vi "DSOpen.vi"(8 "Array":string[](array[string]), 9 "mode":T1(ring), 10 "I/O":enum16{"Input", "Output"}(ring), 11 "Slot":T2(ring)=enum."Dnet1") -> (0 "error Out":errorcluster[](array[cluster]), 3 "connection out":refnum<k13>[](array[refnum]))   [LabVIEW 2011]
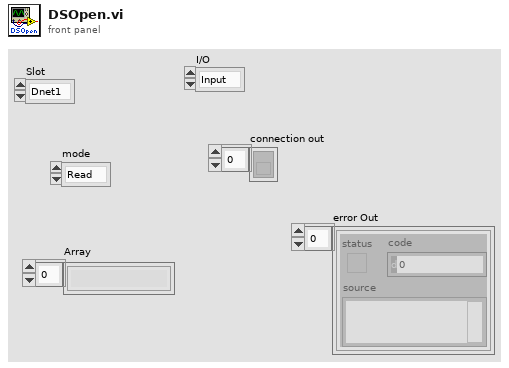
[diagram p1: front panel]
types:
  T1 = enum16{"Read", "Write", "ReadWrite", "BufferedRead", "BufferedReadWrite"}
  T2 = enum16{"OPC Server", "Global", "Dnet1", "Dnet2", "Dnet3", "Ain1", "Ain2", "Aout1", "Din1", "Din2", "Dout1"}
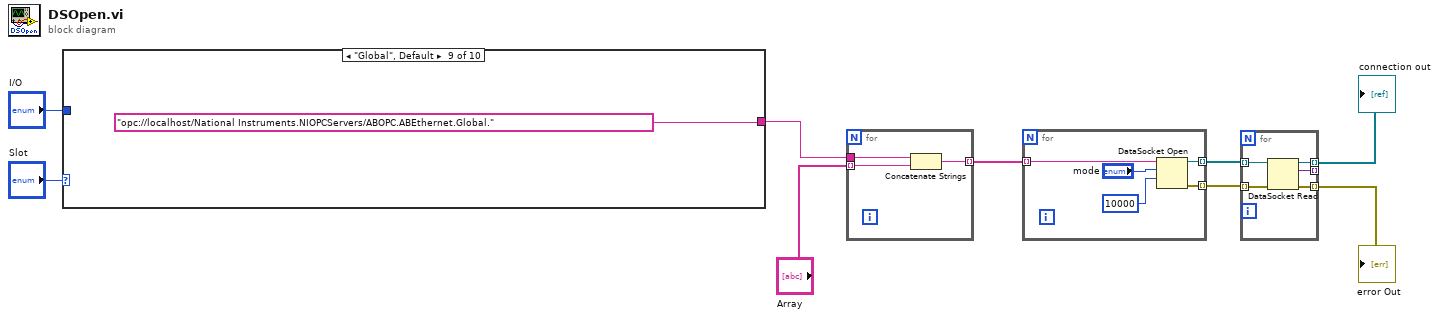
[diagram p0: block diagram]
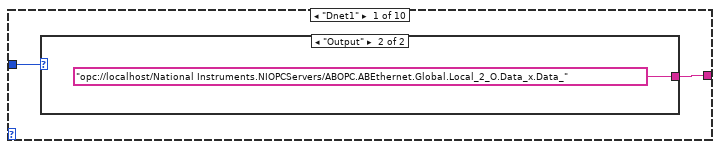
[diagram p2: hidden frame]
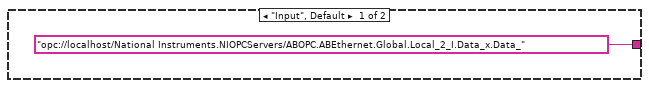
[diagram p3: hidden frame]
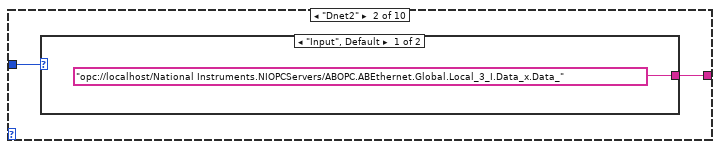
[diagram p4: hidden frame]
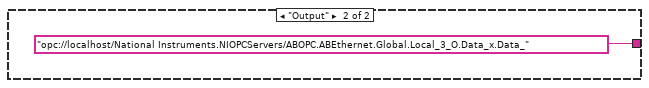
[diagram p5: hidden frame]
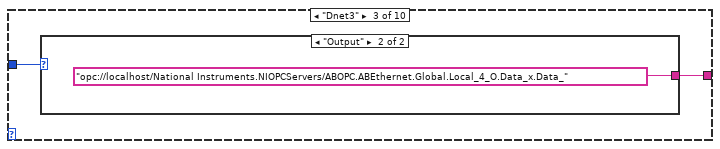
[diagram p6: hidden frame]
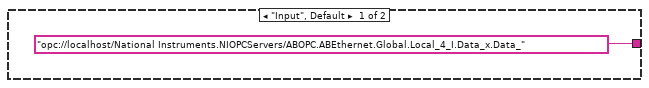
[diagram p7: hidden frame]
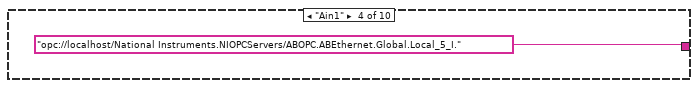
[diagram p8: hidden frame]
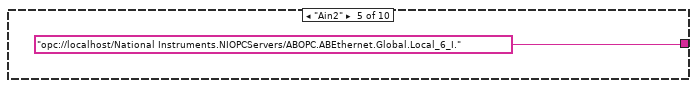
[diagram p9: hidden frame]
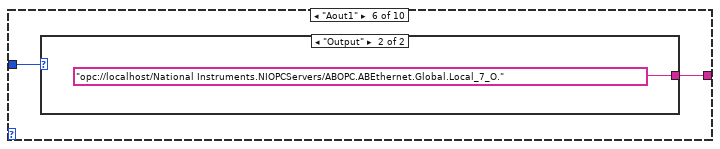
[diagram p10: hidden frame]
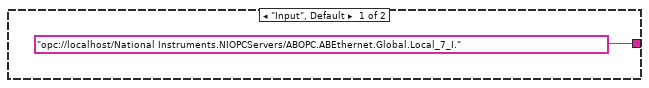
[diagram p11: hidden frame]
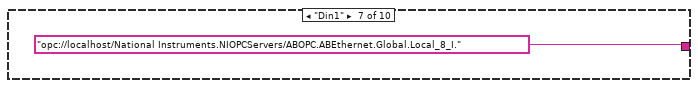
[diagram p12: hidden frame]
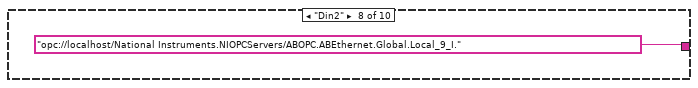
[diagram p13: hidden frame]
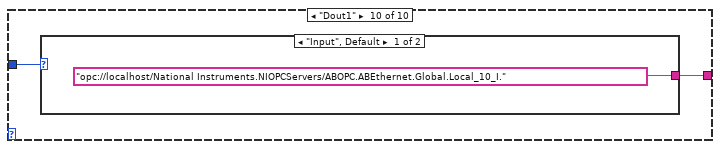
[diagram p14: hidden frame]
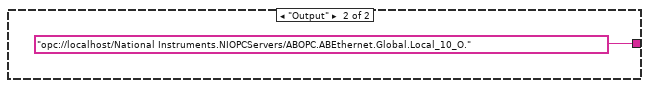
[diagram p15: hidden frame]
diagram:
  n1 = case shown="\"Global\", Default" "Slot" {
    tunnel: "I/O" -> [w11 w15 w19 _ _ w25 _ _ _ w32]
    tunnel: [w10 w14 w18 "opc://localhost/National Instruments.NIOPCServers/ABOPC.ABEthernet.Global.Local_5_I." "opc://localhost/National Instruments.NIOPCServers/ABOPC.ABEthernet.Global.Local_6_I." w24 "opc://localhost/National Instruments.NIOPCServers/ABOPC.ABEthernet.Global.Local_8_I." "opc://localhost/National Instruments.NIOPCServers/ABOPC.ABEthernet.Global.Local_9_I." "opc://localhost/National Instruments.NIOPCServers/ABOPC.ABEthernet.Global." w31] -> w8
    frame "Dnet1" {
      n2 = case shown="\"Output\"" w11 {
        tunnel: ["opc://localhost/National Instruments.NIOPCServers/ABOPC.ABEthernet.Global.Local_2_I.Data_x.Data_" "opc://localhost/National Instruments.NIOPCServers/ABOPC.ABEthernet.Global.Local_2_O.Data_x.Data_"] -> w10
        frame "Input", Default {
        }
        frame "Output" {
        }
      }
    }
    frame "Dnet2" {
      n3 = case shown="\"Input\", Default" w15 {
        tunnel: ["opc://localhost/National Instruments.NIOPCServers/ABOPC.ABEthernet.Global.Local_3_I.Data_x.Data_" "opc://localhost/National Instruments.NIOPCServers/ABOPC.ABEthernet.Global.Local_3_O.Data_x.Data_"] -> w14
        frame "Input", Default {
        }
        frame "Output" {
        }
      }
    }
    frame "Dnet3" {
      n4 = case shown="\"Output\"" w19 {
        tunnel: ["opc://localhost/National Instruments.NIOPCServers/ABOPC.ABEthernet.Global.Local_4_I.Data_x.Data_" "opc://localhost/National Instruments.NIOPCServers/ABOPC.ABEthernet.Global.Local_4_O.Data_x.Data_"] -> w18
        frame "Input", Default {
        }
        frame "Output" {
        }
      }
    }
    frame "Ain1" {
    }
    frame "Ain2" {
    }
    frame "Aout1" {
      n5 = case shown="\"Output\"" w25 {
        tunnel: ["opc://localhost/National Instruments.NIOPCServers/ABOPC.ABEthernet.Global.Local_7_I." "opc://localhost/National Instruments.NIOPCServers/ABOPC.ABEthernet.Global.Local_7_O."] -> w24
        frame "Input", Default {
        }
        frame "Output" {
        }
      }
    }
    frame "Din1" {
    }
    frame "Din2" {
    }
    frame "Global", Default {
    }
    frame "Dout1" {
      n6 = case shown="\"Input\", Default" w32 {
        tunnel: ["opc://localhost/National Instruments.NIOPCServers/ABOPC.ABEthernet.Global.Local_10_I." "opc://localhost/National Instruments.NIOPCServers/ABOPC.ABEthernet.Global.Local_10_O."] -> w31
        frame "Input", Default {
        }
        frame "Output" {
        }
      }
    }
  }
  n7 = for {
    tunnel: w8 -> [w37]
    tunnel: "Array" -> [w36] mode=indexing
    tunnel: [w35] -> w6 mode=indexing
    n8 = Concatenate Strings(w37, w36) -> (w35:string)
  }
  n9 = for {
    tunnel: [w41] -> w5 mode=indexing
    tunnel: [w40] -> w4 mode=indexing
    tunnel: w6 -> [w38] mode=indexing
    n10 = DataSocket Open(9:10000 ("ms timeout (10000)"), 10:"mode", 11:w38) -> (0:w40:errorcluster, 3:w41:refnum<k13>)  [unwired: 1 in]
  }
  n11 = for {
    tunnel: [w47] -> w2 mode=indexing
    tunnel: [w46] -> w1 mode=indexing
    tunnel: w5 -> [w45] mode=indexing
    tunnel: w4 -> [w44] mode=indexing
    tunnel: [w43] -> _ mode=indexing
    n12 = DataSocket Read(8:w44, 11:w45) -> (0:w47:errorcluster, 2:w43:variant, 3:w46:refnum<k13>)  [unwired: 1 in, 6 out]
  }
  "error Out" <- w2
  "connection out" <- w1
